vi "limits_loadSpec.vi"(8 "error in (no error)":errorcluster, 11 "limits file":path) -> (0 "error out":errorcluster, 2 "test limits":T1[](array[typedef]))   [LabVIEW 2019]
uses:
  limits_limitList.ctl
  limits_specs.ctl
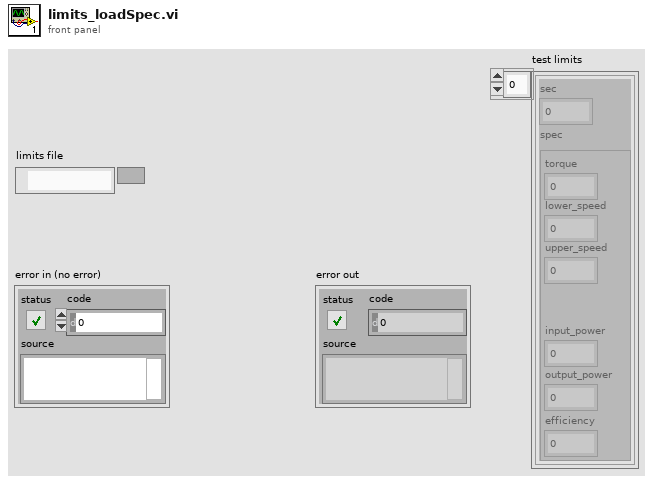
[diagram p1: front panel]
types:
  T1 = typedef "limits_limitList.ctl" = cluster{"sec":i32, "spec":T2}
  T2 = typedef "limits_specs.ctl" = cluster{"torque":dbl, "lower_speed":dbl, "upper_speed":dbl, "input_power":dbl, "output_power":dbl, "efficiency":dbl}
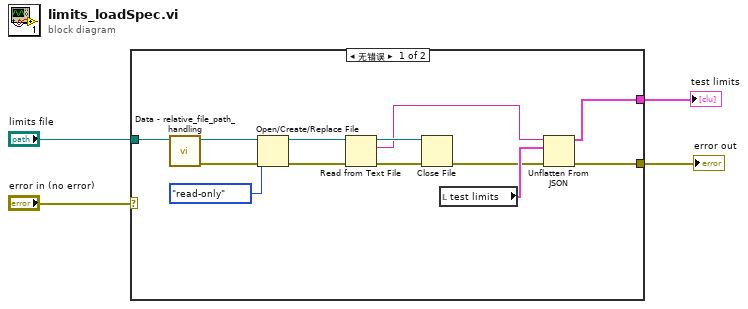
[diagram p0: block diagram]
diagram:
  n1 = case shown="无错误" "error in (no error)" {
    selector: "error in (no error)" -> [_ w18]
    tunnel: "limits file" -> [w17 _]
    tunnel: [w6 w18] -> w3
    tunnel: [w5 _] -> w2
    frame No Error {
      n2 = call "Data - relative_file_path_handling.vi"("path in"=w17) -> ("error out"=w12:errorcluster, "path out"=w15:path)  [unwired: 9 in]
      n3 = Open/Create/Replace File(file path (use dialog)=w15, error in=w12, access (0:read/write)=enum16{"read/write", "read-only", "write-only"}."read-only") -> (refnum out=w14:refnum<file>, error out=w11:errorcluster)  [unwired: 3 in, 1 out]
      n4 = Read from Text File(file (use dialog)=w14, error in=w11) -> (refnum out=w13:refnum<file>, text=w8:string, error out=w10:errorcluster)  [unwired: 2 in, 1 out]
      n5 = Close File(refnum=w13, error in=w10) -> (error out=w9:errorcluster)  [unwired: 1 out]
      n6 = local read "test limits"() -> (w16:T1[])
      n7 = Unflatten From JSON(JSON string=w8, type and defaults=w16, error in (no error)=w9) -> (value=w5:T1[], error out=w6:errorcluster)  [unwired: 4 in]
    }
    frame Error {
    }
  }
  "error out" <- w3
  "test limits" <- w2
